vi "KEITHLEY_2260B.vi"() -> ()   [LabVIEW 2026]
uses:
  <vilib>/Platform/TimedLoop/XDataNode/timing_clust.ctl
  <vilib>/Platform/TimedLoop/XDataNode/nitl_modes.ctl
  <vilib>/Platform/TimedLoop/XDataNode/wakeup.ctl
  <vilib>/Instr/_visa.llb/VISA Configure Serial Port (Instr).vi
  <vilib>/platform/TimedLoop/XDataNode/XDataNode.xnode
  <vilib>/Platform/TimedLoop/XDataNode/XDNodeRunTimeDep.lvlib
panel:
  out "error out":errorcluster
  out "2260B_A":string caption="A"
  in  "Enum":T1(ring)
  in  "2260 COM PORT":refnum<visa-resource-name>
  in  "stop":bool
  out "2260B_module_name":string
  in  "2260B_SET_PWR DSPL":bool caption="PWR DSPL"
  in  "2260B_SET_Lock/Local":bool caption="Lock/Local"
  in  "2260B_SET_Utility":bool caption="Utility"
  in  "2260B_SET_Set":bool caption="Set"
  in  "2260B_SET_OVP/OCP":bool caption="OVP/OCP"
  in  "2260B_SET_Function":bool caption="Function"
  in  "2260B_set_Output":bool caption="Output"
  in  "2260B_set_Current":dbl(knob) caption="Current" scale=0.0..10.0
  in  "2260B_set_voltage":dbl(knob) caption="Voltage" scale=0.0..10.0
  out "2260B_V":string caption="V"
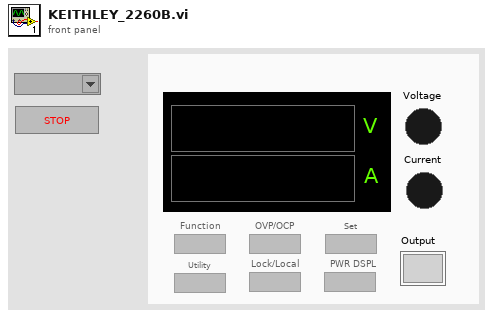
[diagram p1: front panel]
types:
  T1 = enum16{"*IDN?", "MEAS:VOLT?", "MEAS:CURR?", "OUTP?"}
  T2 = typedef "XDNodeRunTimeDep.lvlib/timing_clust.ctl" = cluster{"Expected End [f-1]":u64, "Actual End [f-1]":u64, "Finished Late? [f-1]":bool, "Expected End [i-1]":u64, "Actual End [i-1]":u64, "Finished Late? [i-1]":bool, "Expected Start [i]":u64, "Actual Start [i]":u64, "Expected Start [f]":u64, "Actual Start [f]":u64, "Source Name":string, "Structure Name":string, "Period":i64, "Deadline":i64, "Offset":i64, "Start":i64, "Priority":i32, "Timeout":i32, "Mode":T3, "Wakeup Reason":T4, "Error":errorcluster, "Source Type":string, "Secondary Source Type":string, "Global End Time":u64, "Global Start Time":u64, "Frame Duration":u64, "Iteration Duration":u64, "Assigned CPU":i32, "I/O Scan Engine Mode":u32}
  T3 = typedef "XDNodeRunTimeDep.lvlib/nitl_modes.ctl" = enum32{"No Change", "Process missed periods, maintain original phase", "Discard missed periods, maintain original phase", "Process missed periods, ignore original phase", "Discard missed periods, ignore original phase"}
  T4 = typedef "XDNodeRunTimeDep.lvlib/wakeup.ctl" = enum32{"Normal", "Aborted", "Asynchronous wakeup", "Timing source error", "Timed loop error", "Timeout"}
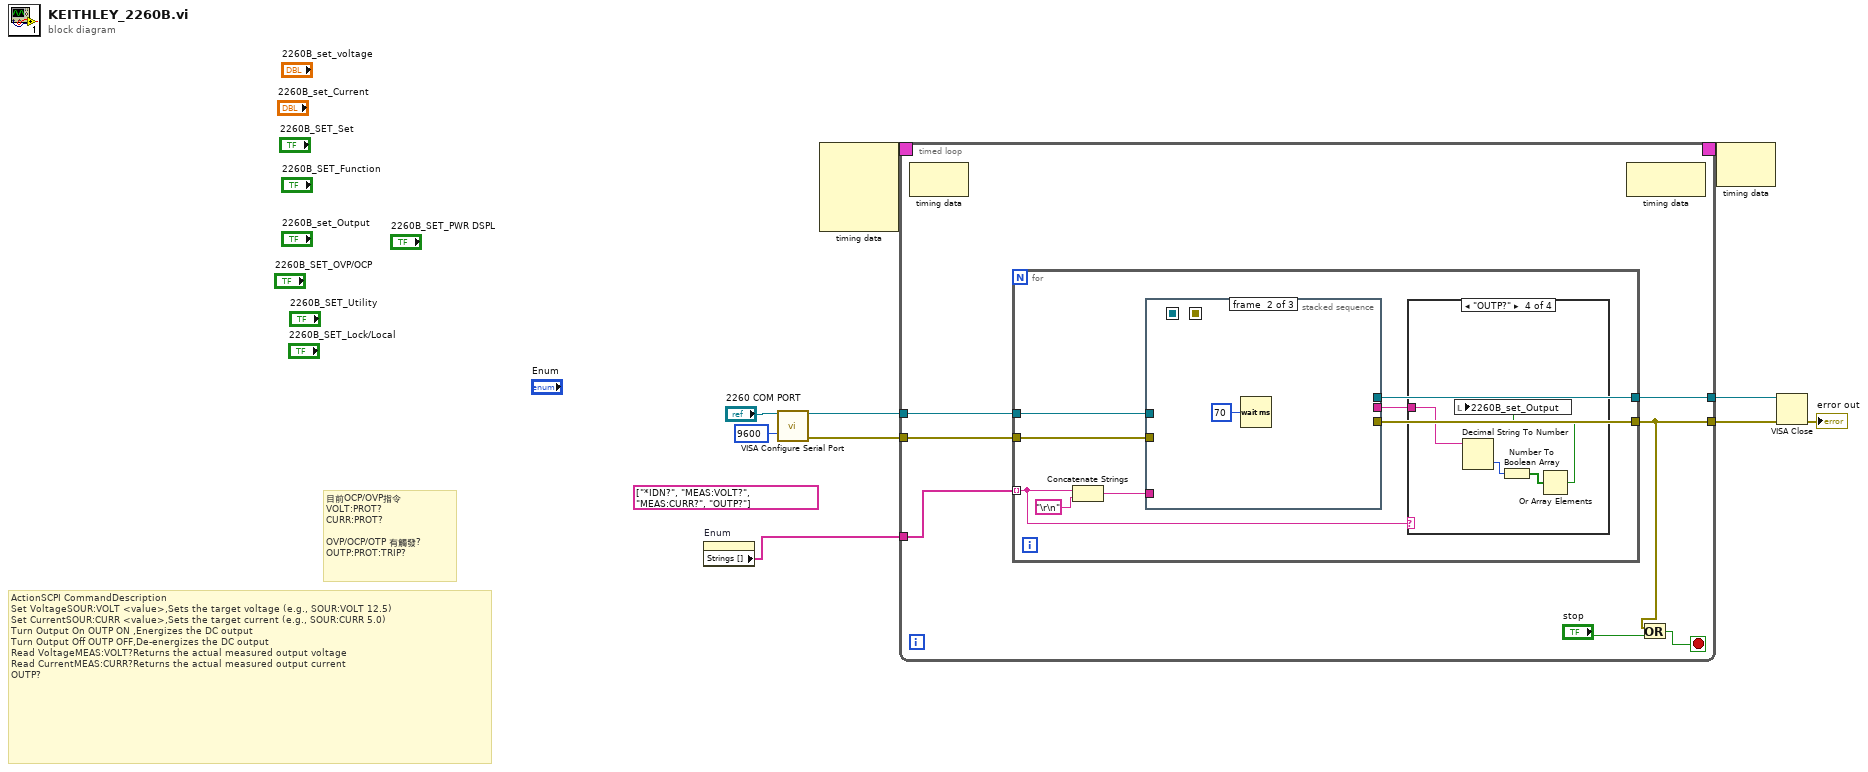
[diagram p0: block diagram]
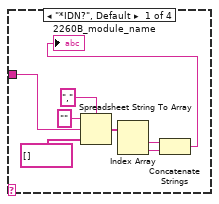
[diagram p2: hidden frame]
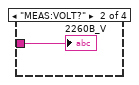
[diagram p3: hidden frame]
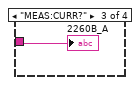
[diagram p4: hidden frame]
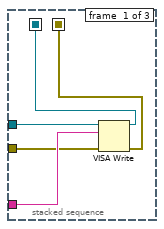
[diagram p5: hidden frame]
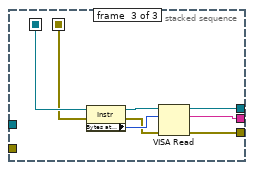
[diagram p6: hidden frame]
diagram:
  (unwired) string[] ["*IDN?", "MEAS:VOLT?", "MEAS:CURR?", "OUTP?"] ("write buffer 2")
  # "目前OCP/OVP指令\nVOLT:PROT?\nCURR:PROT?\n\nOVP/OCP/OTP 有觸發?\nOUTP:PROT:TRIP?"
  # "ActionSCPI CommandDescription\nSet VoltageSOUR:VOLT <value>,Sets the target voltage (e.g., SOUR:VOLT 12.5)\nSet CurrentSOUR:CURR <value>,Sets the target current (e.g., SOUR:CURR 5.0)\nTurn Output On OUTP ON ,Energizes the DC output\nTurn Output Off OUTP OFF,De-energizes the DC output\nRead VoltageMEAS:VOLT?Returns the actual measured output voltage\nRead CurrentMEAS:CURR?Returns the actual measured output current\nOUTP?"
  n1 = property on="Enum" class="Enum (strict)"() -> ("Strings []"=w2:string[])  [unwired: 2 in, 2 out]
  n2 = call-poly "VISA Configure Serial Port"("VISA resource name"="2260 COM PORT", "baud rate (9600)"=u32 9600) -> ("VISA resource name out"=w6:refnum<visa-resource-name>, "error out"=w5:errorcluster)  [unwired: 12 in]
  n3 = node-c288() -> (w10:T2)  [unwired: 4 in]
  n4 = timed-loop {
    timing: w10 -> [_]
    timing-out: [_] -> w9
    tunnel: w6 -> [w17]
    tunnel: w5 -> [w16]
    tunnel: [w15] -> w4
    tunnel: [w12] -> w3
    tunnel: w2 -> [w14]
    stop <- w11 stop-if-true
    n5 = node-c288() -> ()  [unwired: 1 in, 1 out]
    n6 = for {
      tunnel: w14 -> [w21] mode=indexing
      tunnel: w17 -> [w25]
      tunnel: w16 -> [w24]
      tunnel: [w23] -> w15
      tunnel: [w22] -> w12
      n7 = Concatenate Strings(w21, "\r\n") -> (w26:string)
      n8 = stacked-sequence {
        seq-local: [w44 _ _] -> [_ _ w55]
        seq-local: [w42 _ _] -> [_ _ w51]
        tunnel: w26 -> [w46 _ _]
        tunnel: w25 -> [w45 _ _]
        tunnel: w24 -> [w43 _ _]
        tunnel: [_ _ w50] -> w23
        tunnel: [_ _ w49] -> w22
        tunnel: [_ _ w48] -> w20
        frame #0 {
          n9 = VISA Write(VISA resource name=w45, write buffer=w46, error in (no error)=w43) -> (VISA resource name out=w44:refnum<visa-resource-name>, error out=w42:errorcluster)  [unwired: 1 out]
        }
        frame #1 {
          n10 = Wait (ms)(milliseconds to wait=u32 70) -> ()  [unwired: 1 out]
        }
        frame #2 {
          n11 = property class="Instr"(reference=w55, error in=w51) -> (reference out=w54:refnum<visa-resource-name>, error out=w52:errorcluster, "Bytes at Port"=w53:u32)
          n12 = VISA Read(VISA resource name=w54, byte count=w53, error in (no error)=w52) -> (VISA resource name out=w50:refnum<visa-resource-name>, read buffer=w48:string, error out=w49:errorcluster)  [unwired: 1 out]
        }
      }
      n13 = case shown="\"OUTP?\"" w21 {
        tunnel: w20 -> [w29 w36 w37 w41]
        frame "*IDN?", Default {
          n14 = Spreadsheet String To Array(delimiter (Tab)="," ("format string"), format string="", spreadsheet string=w29, array type (2D Dbl)=string[] []) -> (array=w33:string[])
          n15 = Index Array(array=w33) -> (element #1=w34:string, element #2=w35:string)  [unwired: 2 in]
          n16 = Concatenate Strings(w34, w35) -> (→"2260B_module_name":string)
        }
        frame "MEAS:VOLT?" {
          "2260B_V" <- w36
        }
        frame "MEAS:CURR?" {
          "2260B_A" <- w37
        }
        frame "OUTP?" {
          n17 = Decimal String To Number(string=w41) -> (number=w40:i32)  [unwired: 2 in, 1 out]
          n18 = Number To Boolean Array(number=w40) -> (Boolean array=w39:bool[])
          n19 = Or Array Elements(Boolean array=w39) -> (logical OR=w38:bool)
          n20 = local write "2260B_set_Output"(w38) -> ()
        }
      }
    }
    n21 = node-c288() -> ()  [unwired: 1 in, 1 out]
    n22 = Or(x=w12, y="stop") -> (x .or. y?=w11:bool)
  }
  n23 = node-c288(w9) -> ()  [unwired: 1 out]
  n24 = VISA Close(VISA resource name=w4, error in (no error)=w3) -> (error out=→"error out":errorcluster)
